vi "Time offset.vi"(8 "error in (no error)":errorcluster, 10 "scale factor":dbl=1000.0 format="%0.2f", 11 "waveform in":waveform(dbl)) -> (0 "error out":errorcluster, 3 "waveform out":waveform(dbl))   [LabVIEW 2022 SP3]
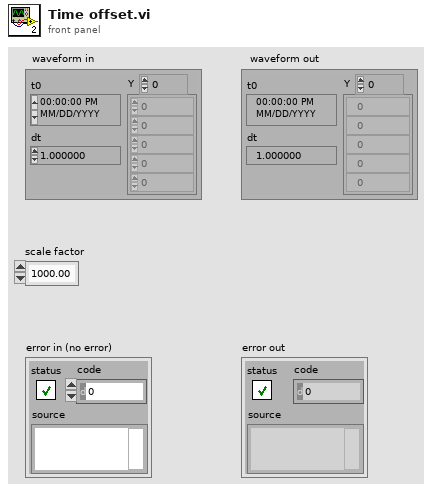
[diagram p1: front panel]
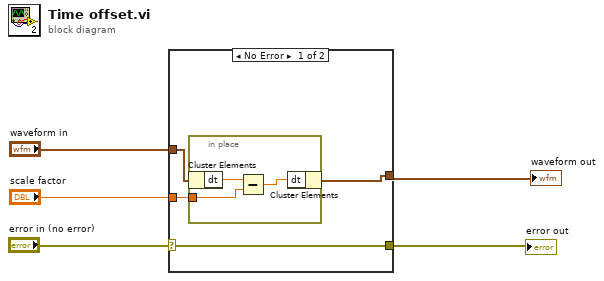
[diagram p0: block diagram]
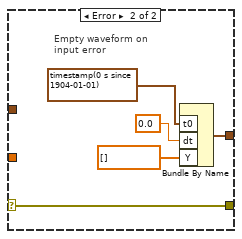
[diagram p2: hidden frame]
diagram:
  n1 = case shown="No Error" "error in (no error)" {
    selector: "error in (no error)" -> [w9 w17]
    tunnel: "waveform in" -> [w8 _]
    tunnel: [w6 w16] -> w1
    tunnel: [w9 w17] -> w4
    tunnel: "scale factor" -> [w7 _]
    frame No Error {
      n2 = in-place {
        in-place-border: w7 -> [w11]
        n3 = in-place-cluster #1(w8) -> ("dt"=w12:dbl)
        n4 = Subtract(x=w12, y=w11) -> (x-y=w10:dbl)
        n5 = in-place-cluster #1("dt"=w10) -> (w6:waveform(dbl))
      }
    }
    frame Error {
      # "Empty waveform on\ninput error"
      n6 = Bundle By Name("t0"=timestamp(0 s since 1904-01-01), "dt"=0.0, "Y"=dbl[] []) -> (w16:waveform(dbl))  [unwired: 1 out]
    }
  }
  "waveform out" <- w1
  "error out" <- w4
